vi "Simulated Data.vi"(8 "error in":errorcluster, 10 "Simulated Data":bool, 11 "Refnum in":refnum<k20>) -> (0 "error out":errorcluster, 3 "Refnum out":refnum<k20>)   [LabVIEW 2016, in "Aurora Stream (NI 6592R) (Host).lvlib"]
uses:
  Aurora Stream (NI 6592R) (Host).lvlib
  Base Bitfile Reference.ctl
  <vilib>/Utility/error.llb/Error Cluster From Error Code.vi
  <vilib>/rvi/errors/niLvFpgaAdjustHostInterfaceError.vi
  <vilib>/rvi/interface/nirviReadWriteControl/nirviReadWriteControl.xnode
  NiFpgaLv.dll
  <vilib>/rvi/interface/Simulation/niFpgaSimulationCallBeginRW.vi
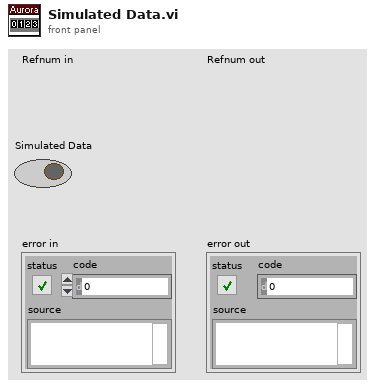
[diagram p1: front panel]
types:
  T1 = typedef "Aurora Stream (NI 6592R) (Host).lvlib/Base Bitfile Reference.ctl" = refnum<k20>
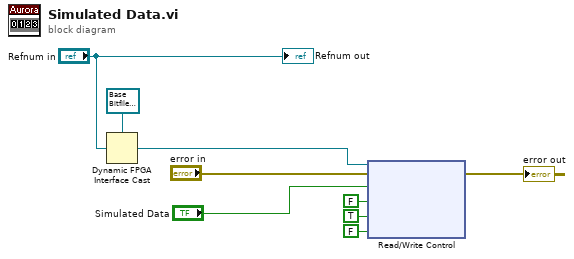
[diagram p0: block diagram]
diagram:
  n1 = Dynamic FPGA Interface Cast(Session In=T1 refnum ("Aurora Sample Project"), Type="Refnum in") -> (Session Out=w5:T1)
  n2 = xnode "Read/Write Control"("FPGA VI Reference In"=w5, "error in"="error in", "Simulated data"="Simulated Data", "Reset"=FALSE, "Reset"=TRUE, "Reset"=FALSE) -> ("error out"=→"error out":errorcluster)  [unwired: 1 out]
  "Refnum out" <- "Refnum in"
